vi "控件测试页.vi"() -> ()   [LabVIEW 2018]
panel:
  in  "布尔 2":bool
  in  "字符串":string
  in  "布尔":bool
  in  "数值 2":dbl
  in  "数值":dbl
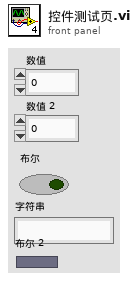
[diagram p1: front panel]
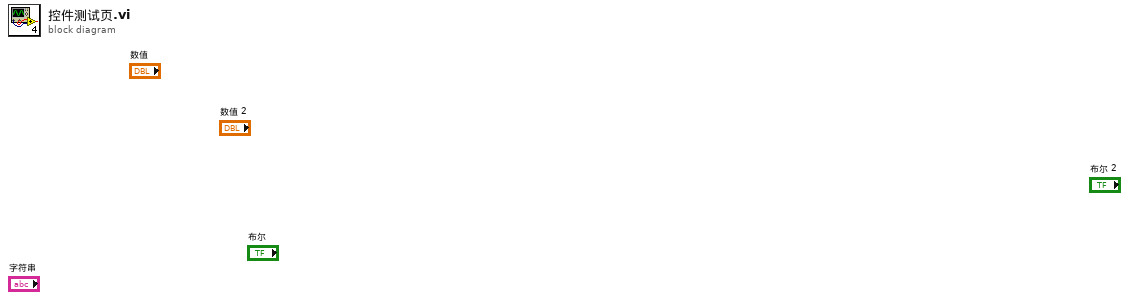
[diagram p0: block diagram]
diagram:
